vi "Manjeo_Cadenas.vi"() -> ()   [LabVIEW 2020]
panel:
  in  "input 1":dbl
  out "output 1":dbl
  out "after substring":string
  out "before substring":string
  out "match substring":string
  out "length":i32
  out "offset past match":i32
  out "concatenated string":string
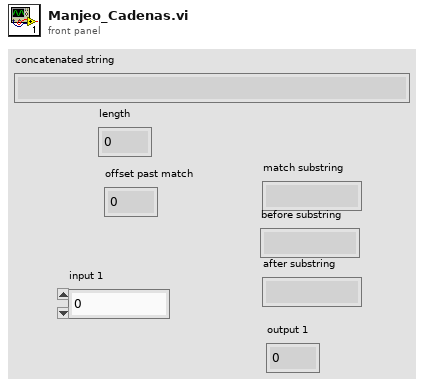
[diagram p1: front panel]
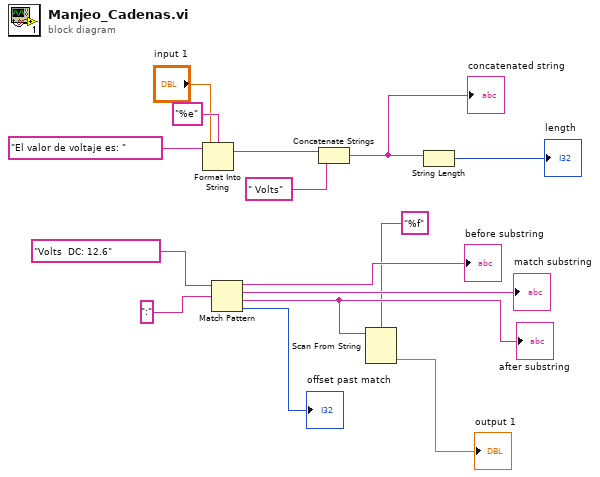
[diagram p0: block diagram]
diagram:
  n1 = Format Into String "Format Into String"(format string="%e", initial string="El valor de voltaje es: ", "input 1") -> (resulting string=w13:string)  [unwired: 1 in, 1 out]
  n2 = Match Pattern(string="Volts  DC: 12.6", regular expression=":") -> (before substring=→"before substring":string, match substring=→"match substring":string, after substring=w4:string, offset past match=→"offset past match":i32)  [unwired: 1 in]
  "after substring" <- w4
  n3 = Concatenate Strings "Concatenate Strings"(w13, " Volts" ("string")) -> (w11:string)
  "concatenated string" <- w11
  n4 = Scan From String "Scan From String"(format string="%f", input string=w4) -> (output 1=→"output 1":dbl)  [unwired: 3 in, 3 out]
  n5 = String Length(string=w11) -> (length=→"length":i32)
